vi "Set XY Accleration.vi"(0 "Gantry In":refnum<k24>, 1 "mm/s":dbl=200.0 format="%#_13g", 3 "error in (no error)":errorcluster) -> (7 "Gantry Out":refnum<k24>, 8 "X":dbl, 10 "error out":errorcluster)   [LabVIEW 2019, in "A3200.lvclass"]
uses:
  A3200.lvclass
  C:/Program Files (x86)/Aerotech/A3200/LabVIEW/2010/Bin/Aerotech.A3200.dll
  Program Files (x86)/Aerotech/A3200/LabVIEW/2010/Bin/Aerotech.A3200.dll
  Drivers/Aerotech A3200/Aerotech VIs.lvlib
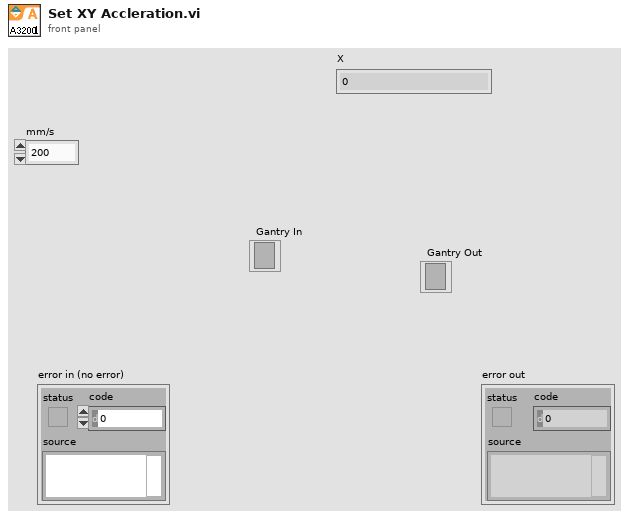
[diagram p1: front panel]
types:
  T1 = cluster{"Status":bool, "Error Code":i32, "Source":string}
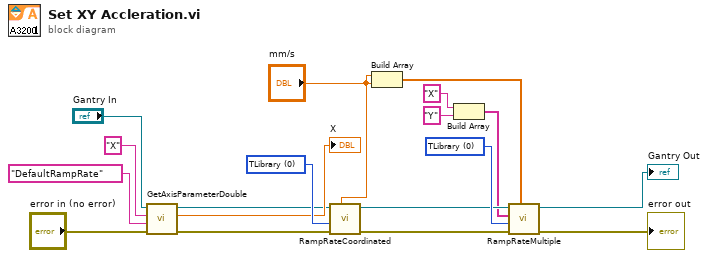
[diagram p0: block diagram]
diagram:
  w16 = 0 items=["TLibrary", "T01", "T02", "T03", "T04", "T05", "T06", "T07", "T08", "T09", "T10", "T11", "T12", "T13", "T14", "T15", "T16", "T17", "T18", "T19", "T20", "T21", "T22", "T23", "T24", "T25", "T26", "T27", "T28", "T29", "T30", "T31"] ("task id")
  w17 = 0 items=["TLibrary", "T01", "T02", "T03", "T04", "T05", "T06", "T07", "T08", "T09", "T10", "T11", "T12", "T13", "T14", "T15", "T16", "T17", "T18", "T19", "T20", "T21", "T22", "T23", "T24", "T25", "T26", "T27", "T28", "T29", "T30", "T31"] ("taskId")
  n1 = call "GetAxisParameterDouble.vi"("error in (no error)"="error in (no error)", "Parameter Name"="DefaultRampRate", "axis name"="X", "controller in"="Gantry In") -> ("error out"=w1:errorcluster, "value"=→"X":dbl, "controller out"=w2:refnum<k24>)  [unwired: 5 in]
  n2 = call "RampRateCoordinated.vi"("ramp rate"="mm/s", "error in (no error)"=w1, "taskId"=w17, "controller in"=w2) -> ("error out"=w8:T1, "controller out"=w15:refnum<k24>)  [unwired: 6 in]
  n3 = Build Array("mm/s", "mm/s") -> (w18:dbl[])
  n4 = Build Array("X", "Y") -> (w12:string[])
  n5 = call "RampRateMultiple.vi"("ramp rates"=w18, "error in (no error)"=w8, "task id"=w16, "axis names"=w12, "controller in"=w15) -> ("error out (no error)"=→"error out":T1, "controller out"=→"Gantry Out":refnum<k24>)  [unwired: 5 in]
